vi "LINC Align Packet.vi"(7 "initial offset":i32, 8 "error in (no error)":errorcluster, 10 "item formats in":T1[](array[typedef])) -> (0 "error out":errorcluster, 2 "item formats out":T1[](array[typedef]))   [LabVIEW 2018, in "STEPkgDriver_LINC.lvlib"]
uses:
  STEPkgDriver_LINC.lvlib
  LINC Format Prototype.ctl
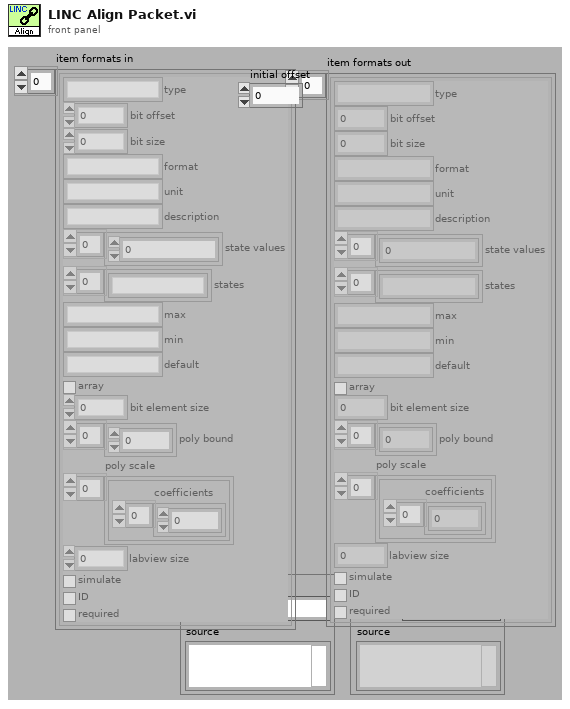
[diagram p1: front panel]
types:
  T1 = typedef "STEPkgDriver_LINC.lvlib/LINC Format Prototype.ctl" = cluster{"type":string, "bit offset":i32, "bit size":i32, "format":string, "unit":string, "description":string, "state values":i64[], "states":string[], "max":string, "min":string, "default":string, "array":bool, "bit element size":i32, "poly bound":dbl[], "poly scale":cluster{"coefficients":dbl[]}[], "labview size":i32, "simulate":bool, "ID":bool, "required":bool}
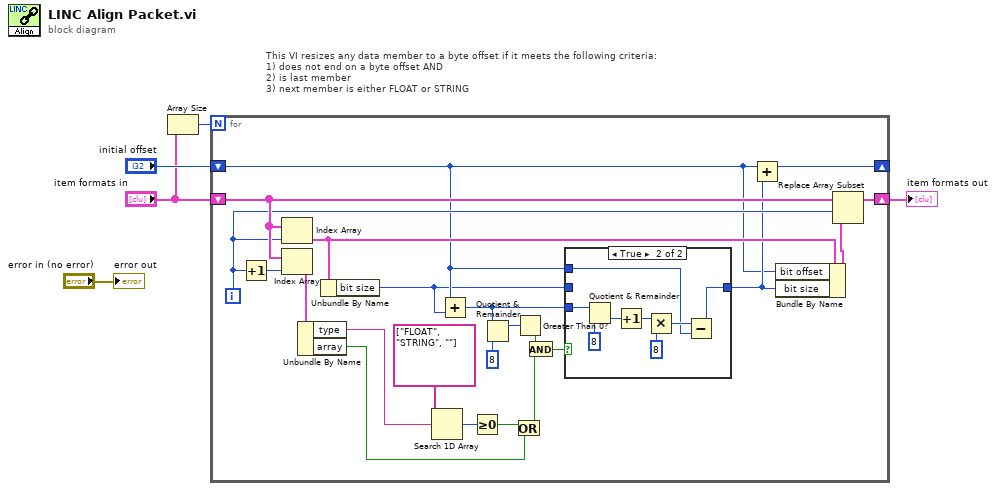
[diagram p0: block diagram]
diagram:
  # "This VI resizes any data member to a byte offset if it meets the following criteria:\n1) does not end on a byte offset AND\n2) is last member\n3) next member is either FLOAT or STRING"
  n1 = Array Size(array="item formats in") -> (size(s)=w5:i32)
  n2 = for {
    N: w5 -> [_]
    shift-right: [w27] -> w2
    shift-left: "item formats in" -> [w26]
    shift-right: [w15] -> _
    shift-left: "initial offset" -> [w7]
    i -> [w25]
    n3 = Increment(x=w25) -> (x+1=w24:i32)
    n4 = Index Array(array=w26, index=w25) -> (element=w22:T1)
    n5 = Index Array(array=w26, index=w24) -> (element=w21:T1)
    n6 = Unbundle By Name(w21) -> ("type"=w19:string, "array"=w16:bool)
    n7 = Unbundle By Name(w22) -> ("bit size"=w6:i32)
    n8 = Search 1D Array(1D array=string[] ["FLOAT", "STRING", ""], element=w19) -> (index of element=w18:i32)  [unwired: 1 in]
    n9 = Add(x=w7, y=w6) -> (x+y=w8:i32)
    n10 = Greater Or Equal To 0?(x=w18) -> (x >= 0?=w17:bool)
    n11 = Quotient & Remainder(x=w8, y=8) -> (x-y*floor(x/y)=w13:i32)  [unwired: 1 out]
    n12 = Or(x=w17, y=w16) -> (x .or. y?=w11:bool)
    n13 = Greater Than 0?(x=w13) -> (x > 0?=w12:bool)
    n14 = And(x=w12, y=w11) -> (x .and. y?=w10:bool)
    n15 = case shown="True" w10 {
      tunnel: w8 -> [_ w33]
      tunnel: [w28 w29] -> w9
      tunnel: w7 -> [_ w30]
      tunnel: w6 -> [w28 _]
      frame False {
      }
      frame True {
        n16 = Quotient & Remainder(x=w33, y=8) -> (floor(x/y)=w32:i32)  [unwired: 1 out]
        n17 = Increment(x=w32) -> (x+1=w36:i32)
        n18 = Multiply(x=w36, y=8) -> (x*y=w31:i32)
        n19 = Subtract(x=w31, y=w30) -> (x-y=w29:i32)
      }
    }
    n20 = Add(x=w7, y=w9) -> (x+y=w15:i32)
    n21 = Bundle By Name(cluster=w22, "bit offset"=w7, "bit size"=w9) -> (w23:T1)
    n22 = Replace Array Subset(array=w26, new element=w23, index=w25) -> (w27:T1[])
  }
  "item formats out" <- w2
  "error out" <- "error in (no error)"
